vi "SetBaseFileName.vi"(8 "error in":errorcluster, 10 "BaseFileName":string, 11 "Datawarehouse in":refnum<class "Datawarehouse.lvclass">) -> (0 "error out":errorcluster, 3 "Datawarehouse out":refnum<class "Datawarehouse.lvclass">)   [LabVIEW 2021, in "ProligentXMLGenerator.lvlib" / "Datawarehouse.lvclass"]
doc: "Base file name used to create the full file name.\n\nThe full file name is composed of a \"Proligent_\" prefix and the \".xml\" extension.\n\nThis valus must not be empty."
uses:
  Datawarehouse.lvclass
  Datawarehouse.lvclass/Datawarehouse.ctl
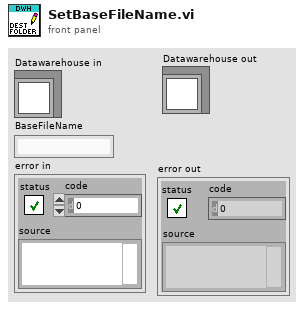
[diagram p1: front panel]
types:
  T1 = typedef "ProligentXMLGenerator.lvlib/Datawarehouse.lvclass/Data.ctl" = cluster{"DestinationFolder":path, "BaseFileName":string, "Document":refnum<k20>, "Defects":refnum<class "Defect.lvclass">[], "TopProcessRuns":refnum<class "ProcessRun.lvclass">[], "ProductUnits":refnum<class "ProductUnit.lvclass">[], "GenerationTime":refnum<class "DateTime.lvclass">, "DataSourceFingerprint":refnum<class "NonEmptyString_448.lvclass">, "IntegrationMetaData":refnum<class "NonEmptyString_2000.lvclass">, "TimeZoneInfoId":string}
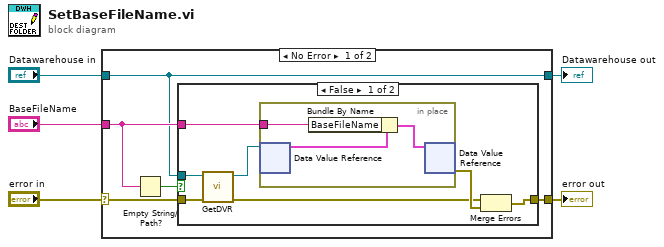
[diagram p0: block diagram]
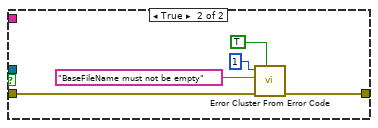
[diagram p2: hidden frame]
diagram:
  n1 = case shown="No Error" "error in" {
    selector: "error in" -> [w10 w26]
    tunnel: "Datawarehouse in" -> [w6 w27]
    tunnel: [w9 w26] -> w3
    tunnel: "BaseFileName" -> [w7 _]
    tunnel: [w6 w27] -> w1
    frame No Error {
      n2 = Empty String/Path?(string/path=w7) -> (empty?=w8:bool)
      n3 = case shown="False" w8 {
        tunnel: w10 -> [w17 w21]
        tunnel: w6 -> [w16 _]
        tunnel: [w15 w24] -> w9
        tunnel: w7 -> [w11 _]
        frame False {
          n4 = call "GetDVR.vi"("error in"=w17, "Datawarehouse"=w16) -> ("error out"=w12:errorcluster, "DVRReference"=w13:refnum<data-value>)  [unwired: 8 in]
          n5 = in-place "In Place Element Structure" {
            in-place-border: w11 -> [w19]
            n6 = in-place-dvr #1(w13) -> (w18:T1)  [unwired: 1 out]
            n7 = Bundle By Name(cluster=w18, "BaseFileName"=w19) -> (w20:T1)
            n8 = in-place-dvr #1(w20) -> (w14:errorcluster)  [unwired: 1 out]
          }
          n9 = Merge Errors(w12, w14) -> (w15:errorcluster)
        }
        frame True {
          n10 = call <vilib>:"Error Cluster From Error Code.vi"("show call chain? (False)"=TRUE, "error in (no error)"=w21, "error message (\"\")"="BaseFileName must not be empty", "error code (0)"=1) -> ("error out"=w24:errorcluster)  [unwired: 5 in]
        }
      }
    }
    frame Error {
    }
  }
  "error out" <- w3
  "Datawarehouse out" <- w1
